vi "getEventUserEventInstance.vi"(8 "error in (no error)":errorcluster, 11 "tcpServer in":refnum<class "TcpServer.lvclass">) -> (0 "error out":errorcluster, 2 "Event":refnum<user-event>, 3 "tcpServer out":refnum<class "TcpServer.lvclass">)   [LabVIEW 2018, in "TcpServer.lvclass"]
doc: "Get the event user event instance."
uses:
  TcpServer.lvclass
  typedef/eventTypeDef.ctl
  TcpServer.lvclass/TcpServer.ctl
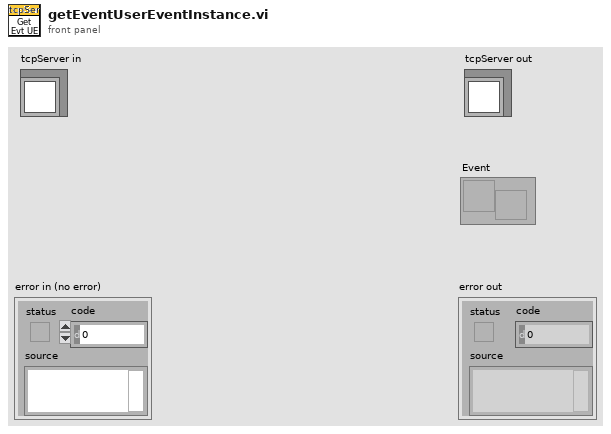
[diagram p1: front panel]
types:
  T1 = typedef "TcpServer.lvclass/userEventsTypeDef.ctl" = cluster{"TcpServer":refnum<user-event>, "Cmd":refnum<user-event>, "CmdStatus":refnum<user-event>, "Event":refnum<user-event>}
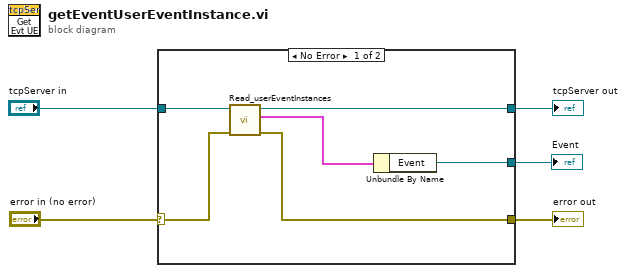
[diagram p0: block diagram]
diagram:
  n1 = case shown="No Error" "error in (no error)" {
    selector: "error in (no error)" -> [w7 w13]
    tunnel: [w6 w13] -> w4
    tunnel: [w10 w12] -> w2
    tunnel: "tcpServer in" -> [w11 w12]
    tunnel: [w8 _] -> w1
    frame No Error {
      n2 = call "Read_userEventInstances.vi"("error in (no error)"=w7, "tcpServer in"=w11) -> ("error out"=w6:errorcluster, "UserEvents"=w9:T1, "tcpServer out"=w10:refnum<class "TcpServer.lvclass">)  [unwired: 7 in]
      n3 = Unbundle By Name(w9) -> ("Event"=w8:refnum<user-event>)
    }
    frame Error {
    }
  }
  "error out" <- w4
  "tcpServer out" <- w2
  "Event" <- w1
